vi "NavbalLabVIEW(15-5-28.vi"() -> ()   [LabVIEW 2012] (continued)
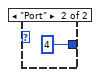
[diagram p2: hidden frame]
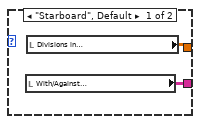
[diagram p4: hidden frame]
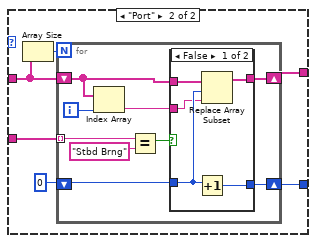
[diagram p6: hidden frame]
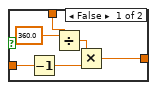
[diagram p10: hidden frame]
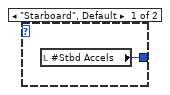
[diagram p11: hidden frame]
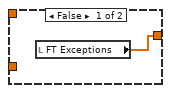
[diagram p12: hidden frame]
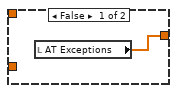
[diagram p13: hidden frame]
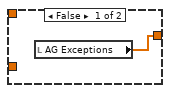
[diagram p14: hidden frame]
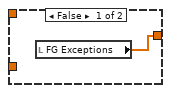
[diagram p15: hidden frame]
                  n2652 = Select(t=w3012, s=w3013, f="  ") -> (s? t:f=w3022:string)
                  n2653 = Number To Fractional String(number=w3057, precision (6)=i16 3) -> (F-format string=w3055:string[][])  [unwired: 2 in]
                  n2654 = Build Array(w3052, w3052, w3052, w3052) -> (w3054:string[])
                  n2655 = Select(t=w3044, s=w3036, f=w3020) -> (s? t:f=w3047:string)
                  n2656 = Select(t=w3044, s=w3037, f=w3022) -> (s? t:f=w3046:string)
                  n2657 = Select(t=w3044, s=w3038, f=w3024) -> (s? t:f=w3045:string)
                  n2658 = Insert Into Array(array=w3055, index (row)=1, new element=w3054) -> (w3051:string[][])  [unwired: 1 in]
                  n2659 = Replace Array Subset(array=w3051, new element=w3052, index (row)=3 ("disabled index (row)"), index (col)=0 ("disabled index (col)")) -> (w3042:string[][])
                  n2660 = Build Array(w3047, "  ", w3046, w3045) -> (w3043:string[])
                  n2661 = Insert Into Array(array=w3042, index (col)=4 ("disabled index (col)"), new element=w3043) -> (w3003:string[][])  [unwired: 1 in]
                  n2662 = property on="Aft Generator Balance Plane Split Options" class="MCListbox (strict)"("ItemNames"=w3003) -> ()  [unwired: 2 in, 2 out]
                  "AG Correction 1" <- w2995
                  "AG Correction 2B" <- w2994
                  "AG Correction 2A" <- w2993
                }
                frame 3 {
                  w3081 = 3 ("disabled index (col)")
                  w3091 = 3 ("disabled index (col)")
                  w3108 = 3 ("disabled index (col)")
                  w3121 = "Occupied!  "
                  w3129 = "  "
                  # "List box formatting"
                  n2663 = Build Array "Mass, angle, loc"(w3075, w3074, w3077) -> (w3139:T3)
                  n2664 = Build Array "Mass,angle, loc"(w3073, w3141, w3078) -> (w3140:T3)
                  n2665 = Build Array (concatenate)(w3140, w3139) -> (w3138:T3)
                  n2666 = Build Array "Percent,mass,angle,location"(w3142, w3070, w3143, w3079) -> (w3135:T3)
                  n2667 = Decrement(x=w3078) -> (x-1=w3116:dbl)
                  n2668 = Decrement(x=w3079) -> (x-1=w3115:dbl)
                  n2669 = Decrement(x=w3077) -> (x-1=w3117:dbl)
                  n2670 = Multiply(x=w3116, y=w3068) -> (x*y=w3090:dbl)
                  n2671 = Multiply(x=w3115, y=w3068) -> (x*y=w3080:dbl)
                  n2672 = Multiply(x=w3117, y=w3068) -> (x*y=w3109:dbl)
                  n2673 = Build Array (concatenate) "Percent"(w3137, w3138) -> (w3133:T3)
                  n2674 = Index Array(array=w3111, index (row)=w3080, index (col)=w3081) -> (element=w3112:bool)
                  n2675 = Index Array(array=w3111, index (row)=w3090, index (col)=w3091) -> (element=w3113:bool)
                  n2676 = Index Array(array=w3111, index (row)=w3109, index (col)=w3108) -> (element=w3114:bool)
                  n2677 = Index Array(array=w3076, index (row)=w3090, index (col)=w3091) -> (element=w3092:dbl)
                  n2678 = Index Array(array=w3076, index (row)=w3109, index (col)=w3108) -> (element=w3105:dbl)
                  n2679 = Index Array(array=w3076, index (row)=w3080, index (col)=w3081) -> (element=w3087:dbl)
                  n2680 = Greater Than 0?(x=w3092) -> (x > 0?=w3089:bool)
                  n2681 = Greater Than 0?(x=w3105) -> (x > 0?=w3106:bool)
                  n2682 = Greater Than 0?(x=w3087) -> (x > 0?=w3083:bool)
                  n2683 = Number To Fractional String(number=w3092, precision (6)=i16 1) -> (F-format string=w3093:string)  [unwired: 2 in]
                  n2684 = Number To Fractional String(number=w3105, precision (6)=i16 1) -> (F-format string=w3104:string)  [unwired: 2 in]
                  n2685 = Number To Fractional String(number=w3087, precision (6)=i16 1) -> (F-format string=w3086:string)  [unwired: 2 in]
                  n2686 = Concatenate Strings(w3093, " wt in hole") -> (w3088:string)
                  n2687 = Concatenate Strings(w3104, " wt in hole") -> (w3102:string)
                  n2688 = Concatenate Strings(w3086, " wt in hole") -> (w3082:string)
                  n2689 = Build Array (concatenate)(w3135, w3133) -> (w3134:T3)
                  n2690 = Select(t=w3082, s=w3083, f="  ") -> (s? t:f=w3096:string)
                  n2691 = Select(t=w3102, s=w3106, f="  ") -> (s? t:f=w3100:string)
                  n2692 = Select(t=w3088, s=w3089, f="  ") -> (s? t:f=w3098:string)
                  n2693 = Number To Fractional String(number=w3134, precision (6)=i16 3) -> (F-format string=w3132:string[][])  [unwired: 2 in]
                  n2694 = Build Array(w3129, w3129, w3129, w3129) -> (w3131:string[])
                  n2695 = Select(t=w3121, s=w3112, f=w3096) -> (s? t:f=w3124:string)
                  n2696 = Select(t=w3121, s=w3113, f=w3098) -> (s? t:f=w3123:string)
                  n2697 = Select(t=w3121, s=w3114, f=w3100) -> (s? t:f=w3122:string)
                  n2698 = Insert Into Array(array=w3132, index (row)=1, new element=w3131) -> (w3128:string[][])  [unwired: 1 in]
                  n2699 = Replace Array Subset(array=w3128, new element=w3129, index (row)=3 ("disabled index (row)"), index (col)=0 ("disabled index (col)")) -> (w3119:string[][])
                  n2700 = Build Array(w3124, "  ", w3123, w3122) -> (w3120:string[])
                  n2701 = Insert Into Array(array=w3119, index (col)=4 ("disabled index (col)"), new element=w3120) -> (w3118:string[][])  [unwired: 1 in]
                  n2702 = property on="Fwd Generator Balance Plane Split Options" class="MCListbox (strict)"("ItemNames"=w3118) -> ()  [unwired: 2 in, 2 out]
                  "FG Correction 1" <- w3069
                  "FG Correction 2A" <- w3072
                  "FG Correction 2B" <- w3071
                }
              }
            }
            "2wt-Exceptions" <- w2654
          }
        }
        n2703 = local read "AT Exceptions"() -> (w621:csg[])
        n2704 = local read "2wt-Exceptions"() -> (w620:csg[])
        n2705 = case shown="True" "Omit AT" {
          tunnel: w621 -> [_ w839]
          tunnel: w620 -> [_ w837]
          tunnel: [w833 w834] -> w619
          frame False {
            n2706 = local read "AT Exceptions"() -> (w833:csg[])
          }
          frame True {
            n2707 = Index Array(array=w837, index=0) -> (element=w835:csg)
            n2708 = Insert Into Array(array=w839, index=0, new element=w835) -> (w834:csg[])
          }
        }
        "AT Exceptions" <- w619
        n2709 = local read "FT Exceptions"() -> (w615:csg[])
        n2710 = local read "2wt-Exceptions"() -> (w616:csg[])
        n2711 = case shown="True" "Omit FT" {
          tunnel: w615 -> [_ w832]
          tunnel: w616 -> [_ w830]
          tunnel: [w826 w827] -> w617
          frame False {
            n2712 = local read "FT Exceptions"() -> (w826:csg[])
          }
          frame True {
            n2713 = Index Array(array=w830, index=1) -> (element=w828:csg)
            n2714 = Insert Into Array(array=w832, index=0, new element=w828) -> (w827:csg[])
          }
        }
        "FT Exceptions" <- w617
        n2715 = local read "AG Exceptions"() -> (w623:csg[])
        n2716 = local read "2wt-Exceptions"() -> (w624:csg[])
        n2717 = case shown="True" "Omit AG" {
          tunnel: w623 -> [_ w846]
          tunnel: w624 -> [_ w844]
          tunnel: [w840 w841] -> w625
          frame False {
            n2718 = local read "AG Exceptions"() -> (w840:csg[])
          }
          frame True {
            n2719 = Index Array(array=w844, index=2) -> (element=w842:csg)
            n2720 = Insert Into Array(array=w846, index=0, new element=w842) -> (w841:csg[])
          }
        }
        "AG Exceptions" <- w625
        n2721 = local read "FG Exceptions"() -> (w628:csg[])
        n2722 = local read "2wt-Exceptions"() -> (w627:csg[])
        n2723 = case shown="True" "Omit FG" {
          tunnel: w628 -> [_ w853]
          tunnel: w627 -> [_ w851]
          tunnel: [w847 w848] -> w626
          frame False {
            n2724 = local read "FG Exceptions"() -> (w847:csg[])
          }
          frame True {
            n2725 = Index Array(array=w851, index=3) -> (element=w849:csg)
            n2726 = Insert Into Array(array=w853, index=0, new element=w849) -> (w848:csg[])
          }
        }
        "FG Exceptions" <- w626
        n2727 = local read "Divisions in\nEach Plane"() -> (w636:T3)
        n2728 = local read "1st Available"() -> (w650:bool)
        n2729 = local read "2nd Available"() -> (w649:bool)
        n2730 = local read "3rd Available"() -> (w648:bool)
        n2731 = local read "4th Available"() -> (w647:bool)
        n2732 = case shown="True" w650 {
          tunnel: w636 -> [_ w1024]
          frame False {
          }
          frame True {
            n2733 = invoke on="Aft Turbine Balance Plane Split Options" class="MCListbox (strict)" method="Get DblClk Row"() -> ("Get Double-clicked Row"=w1025:i32)  [unwired: 3 in, 2 out]
            n2734 = Index Array(array=w1024, index (row)=0, index (col)=0 ("disabled index (col)")) -> (element=w1022:dbl)
            n2735 = case shown="2" w1025 {
              tunnel: w1022 -> [_ w1026 w1053]
              frame -2, Default {
                # "-2 is the variable value when no box is currently double clicked"
              }
              frame 0 {
                w1030 = 360.0 ("x")
                w1042 = 0 ("disabled index (col)")
                w1046 = 0 ("disabled index (col)")
                # "Update Pending weights Boolean Array\nwith selected split's locations"
                # "Update Inputs for Prediction tab\nto reflect selected weight split"
                # "Pull mass, Phase, and Location Data\nfrom listbox's array"
                # "Single Mass Option Selected"
                n2736 = local read "AT Correction 1"() -> (w1040:cdb)
                n2737 = Complex To Polar(r * e^(i*theta)=w1040) -> (r=w1039:dbl, theta=w1027:dbl)
                n2738 = Divide(x=w1027, y=3.141592653589793) -> (x/y=w1038:dbl)
                n2739 = local read "Correction Mag"() -> (w1047:T3)
                n2740 = Multiply ("Multiply.vi")(x=180.0, y=w1038) -> (x*y=w1033:dbl)
                n2741 = Add ("Add.vi")(x=w1033, y=w1030) -> (x+y=w1034:dbl)
                n2742 = Greater Than 0?(x=w1033) -> (x > 0?=w1035:bool)
                n2743 = Select(t=w1033, s=w1035, f=w1034) -> (s? t:f=w1032:dbl)
                n2744 = Divide(x=w1026, y=w1030) -> (x/y=w1031:dbl)
                n2745 = Replace Array Subset(array=w1047, new element=w1039, index (row)=w1046, index (col)=w1046) -> (w1045:T3)
                n2746 = Multiply ("Multiply.vi")(x=w1032, y=w1031) -> (x*y=w1029:dbl)
                n2747 = Increment(x=w1029) -> (x+1=w1028:dbl)
                n2748 = local read "Correction Loc"() -> (w1044:T3)
                n2749 = local write "Correction Mag"(w1045) -> ()
                n2750 = Replace Array Subset(array=w1044, new element=w1028, index (row)=w1042, index (col)=w1042) -> (w1043:T3)
                n2751 = local write "Correction Loc"(w1043) -> ()
                n2752 = property on="Aft Turbine Balance Plane Split Options" class="MCListbox (strict)"("SelColor"=u32 40727) -> ()  [unwired: 2 in, 2 out]
              }
              frame 2 {
                w1052 = 360.0 ("x")
                w1066 = 0 ("disabled index (col)")
                w1070 = 0 ("disabled index (col)")
                n2753 = local read "AT Correction 2A"() -> (w1048:cdb)
                n2754 = local read "AT Correction 2B"() -> (w1049:cdb)
                n2755 = local read "Correction Mag"() -> (w1071:T3)
                n2756 = Add ("Add.vi")(x=w1048, y=w1049) -> (x+y=w1065:cdb)
                n2757 = Complex To Polar ("Complex To Polar.vi")(r * e^(i*theta)=w1065) -> (r=w1064:dbl, theta=w1060:dbl)
                n2758 = Divide(x=w1060, y=3.141592653589793) -> (x/y=w1063:dbl)
                n2759 = Replace Array Subset(array=w1071, new element=w1064, index (row)=w1070, index (col)=w1070) -> (w1069:T3)
                n2760 = local write "Correction Mag"(w1069) -> ()
                n2761 = Multiply ("Multiply.vi")(x=180.0, y=w1063) -> (x*y=w1056:dbl)
                n2762 = local read "Correction Loc"() -> (w1068:T3)
                n2763 = Add ("Add.vi")(x=w1056, y=w1052) -> (x+y=w1057:dbl)
                n2764 = Greater Than 0?(x=w1056) -> (x > 0?=w1058:bool)
                n2765 = Select(t=w1056, s=w1058, f=w1057) -> (s? t:f=w1055:dbl)
                n2766 = Divide(x=w1053, y=w1052) -> (x/y=w1054:dbl)
                n2767 = Multiply ("Multiply.vi")(x=w1055, y=w1054) -> (x*y=w1051:dbl)
                n2768 = Increment(x=w1051) -> (x+1=w1050:dbl)
                n2769 = Replace Array Subset(array=w1068, new element=w1050, index (row)=w1066, index (col)=w1066) -> (w1067:T3)
                n2770 = local write "Correction Loc"(w1067) -> ()
                n2771 = property on="Aft Turbine Balance Plane Split Options" class="MCListbox (strict)"("SelColor"=u32 40727) -> ()  [unwired: 2 in, 2 out]
              }
            }
          }
        }
        n2772 = case shown="True" w649 {
          tunnel: w636 -> [_ w1073]
          frame False {
          }
          frame True {
            n2773 = invoke on="Fwd Turbine Balance Plane Split Options" class="MCListbox (strict)" method="Get DblClk Row"() -> ("Get Double-clicked Row"=w1076:i32)  [unwired: 3 in, 2 out]
            n2774 = Index Array(array=w1073, index (row)=1, index (col)=0 ("disabled index (col)")) -> (element=w1072:dbl)
            n2775 = case shown="0" w1076 {
              tunnel: w1072 -> [_ w1078 w1103]
              frame -2, Default {
              }
              frame 0 {
                w1084 = 360.0 ("x")
                n2776 = local read "FT Correction 1"() -> (w1082:cdb)
                n2777 = Complex To Polar(r * e^(i*theta)=w1082) -> (r=w1081:dbl, theta=w1077:dbl)
                n2778 = Divide(x=w1077, y=3.141592653589793) -> (x/y=w1092:dbl)
                n2779 = Multiply ("Multiply.vi")(x=180.0, y=w1092) -> (x*y=w1087:dbl)
                n2780 = Add ("Add.vi")(x=w1087, y=w1084) -> (x+y=w1088:dbl)
                n2781 = Divide(x=w1078, y=w1084) -> (x/y=w1085:dbl)
                n2782 = Greater Than 0?(x=w1087) -> (x > 0?=w1089:bool)
                n2783 = Select(t=w1087, s=w1089, f=w1088) -> (s? t:f=w1086:dbl)
                n2784 = local read "Correction Mag"() -> (w1100:T3)
                n2785 = local read "Correction Loc"() -> (w1097:T3)
                n2786 = Multiply ("Multiply.vi")(x=w1086, y=w1085) -> (x*y=w1083:dbl)
                n2787 = Increment(x=w1083) -> (x+1=w1079:dbl)
                n2788 = Replace Array Subset(array=w1097, new element=w1079, index (row)=1 ("disabled index (row)"), index (col)=0 ("disabled index (col)")) -> (w1096:T3)
                n2789 = Replace Array Subset(array=w1100, new element=w1081, index (row)=1 ("disabled index (row)"), index (col)=0 ("disabled index (col)")) -> (w1098:T3)
                n2790 = local write "Correction Loc"(w1096) -> ()
                n2791 = local write "Correction Mag"(w1098) -> ()
                n2792 = property on="Fwd Turbine Balance Plane Split Options" class="MCListbox (strict)"("SelColor"=u32 40727) -> ()  [unwired: 2 in, 2 out]
              }
              frame 2 {
                w1106 = 360.0 ("x")
                n2793 = local read "FT Correction 2A"() -> (w1102:cdb)
                n2794 = local read "FT Correction 2B"() -> (w1101:cdb)
                n2795 = Add(x=w1102, y=w1101) -> (x+y=w1120:cdb)
                n2796 = Complex To Polar(r * e^(i*theta)=w1120) -> (r=w1119:dbl, theta=w1115:dbl)
                n2797 = local read "Correction Mag"() -> (w1126:T3)
                n2798 = Divide(x=w1115, y=3.141592653589793) -> (x/y=w1118:dbl)
                n2799 = Multiply ("Multiply.vi")(x=180.0, y=w1118) -> (x*y=w1109:dbl)
                n2800 = local read "Correction Loc"() -> (w1123:T3)
                n2801 = Add(x=w1109, y=w1106) -> (x+y=w1110:dbl)
                n2802 = Replace Array Subset(array=w1126, new element=w1119, index (row)=1 ("disabled index (row)"), index (col)=0 ("disabled index (col)")) -> (w1124:T3)
                n2803 = Greater Than 0?(x=w1109) -> (x > 0?=w1111:bool)
                n2804 = local write "Correction Mag"(w1124) -> ()
                n2805 = Select(t=w1109, s=w1111, f=w1110) -> (s? t:f=w1105:dbl)
                n2806 = Divide(x=w1103, y=w1106) -> (x/y=w1107:dbl)
                n2807 = Multiply ("Multiply.vi")(x=w1105, y=w1107) -> (x*y=w1108:dbl)
                n2808 = Increment(x=w1108) -> (x+1=w1104:dbl)
                n2809 = Replace Array Subset(array=w1123, new element=w1104, index (row)=1 ("disabled index (row)"), index (col)=0 ("disabled index (col)")) -> (w1122:T3)
                n2810 = local write "Correction Loc"(w1122) -> ()
                n2811 = property on="Fwd Turbine Balance Plane Split Options" class="MCListbox (strict)"("SelColor"=u32 40727) -> ()  [unwired: 2 in, 2 out]
              }
            }
          }
        }
        n2812 = case shown="True" w648 {
          tunnel: w636 -> [_ w1128]
          frame False {
          }
          frame True {
            n2813 = invoke on="Aft Generator Balance Plane Split Options" class="MCListbox (strict)" method="Get DblClk Row"() -> ("Get Double-clicked Row"=w1131:i32)  [unwired: 3 in, 2 out]
            n2814 = Index Array(array=w1128, index (row)=2, index (col)=0 ("disabled index (col)")) -> (element=w1127:dbl)
            n2815 = case shown="2" w1131 {
              tunnel: w1127 -> [_ w1133 w1157]
              frame -2, Default {
              }
              frame 0 {
                w1143 = 360.0 ("x")
                n2816 = local read "AG Correction 1"() -> (w1146:cdb)
                n2817 = Complex To Polar(r * e^(i*theta)=w1146) -> (r=w1145:dbl, theta=w1134:dbl)
                n2818 = Divide(x=w1134, y=3.141592653589793) -> (x/y=w1135:dbl)
                n2819 = Multiply ("Multiply.vi")(x=180.0, y=w1135) -> (x*y=w1140:dbl)
                n2820 = Greater Than 0?(x=w1140) -> (x > 0?=w1138:bool)
                n2821 = local read "Correction Mag"() -> (w1155:T3)
                n2822 = Add ("Add.vi")(x=w1140, y=w1143) -> (x+y=w1139:dbl)
                n2823 = Select(t=w1140, s=w1138, f=w1139) -> (s? t:f=w1141:dbl)
                n2824 = Divide(x=w1133, y=w1143) -> (x/y=w1142:dbl)
                n2825 = Multiply ("Multiply.vi")(x=w1141, y=w1142) -> (x*y=w1144:dbl)
                n2826 = Increment(x=w1144) -> (x+1=w1132:dbl)
                n2827 = Replace Array Subset(array=w1155, new element=w1145, index (row)=2 ("disabled index (row)"), index (col)=0 ("disabled index (col)")) -> (w1153:T3)
                n2828 = local read "Correction Loc"() -> (w1152:T3)
                n2829 = local write "Correction Mag"(w1153) -> ()
                n2830 = Replace Array Subset(array=w1152, new element=w1132, index (row)=2 ("disabled index (row)"), index (col)=0 ("disabled index (col)")) -> (w1151:T3)
                n2831 = local write "Correction Loc"(w1151) -> ()
                n2832 = property on="Aft Generator Balance Plane Split Options" class="MCListbox (strict)"("SelColor"=u32 40727) -> ()  [unwired: 2 in, 2 out]
              }
              frame 2 {
                w1156 = 360.0 ("x")
                n2833 = local read "AG Correction 2A"() -> (w1159:cdb)
                n2834 = local read "AG Correction 2B"() -> (w1158:cdb)
                n2835 = Add(x=w1159, y=w1158) -> (x+y=w1175:cdb)
                n2836 = Complex To Polar(r * e^(i*theta)=w1175) -> (r=w1174:dbl, theta=w1170:dbl)
                n2837 = local read "Correction Mag"() -> (w1181:T3)
                n2838 = Divide(x=w1170, y=3.141592653589793) -> (x/y=w1173:dbl)
                n2839 = Multiply ("Multiply.vi")(x=180.0, y=w1173) -> (x*y=w1164:dbl)
                n2840 = Add(x=w1164, y=w1156) -> (x+y=w1165:dbl)
                n2841 = Greater Than 0?(x=w1164) -> (x > 0?=w1166:bool)
                n2842 = local read "Correction Loc"() -> (w1178:T3)
                n2843 = Select(t=w1164, s=w1166, f=w1165) -> (s? t:f=w1161:dbl)
                n2844 = Replace Array Subset(array=w1181, new element=w1174, index (row)=2 ("disabled index (row)"), index (col)=0 ("disabled index (col)")) -> (w1179:T3)
                n2845 = Divide(x=w1157, y=w1156) -> (x/y=w1163:dbl)
                n2846 = local write "Correction Mag"(w1179) -> ()
                n2847 = Multiply ("Multiply.vi")(x=w1161, y=w1163) -> (x*y=w1162:dbl)
                n2848 = Increment(x=w1162) -> (x+1=w1160:dbl)
                n2849 = Replace Array Subset(array=w1178, new element=w1160, index (row)=2 ("disabled index (row)"), index (col)=0 ("disabled index (col)")) -> (w1177:T3)
                n2850 = local write "Correction Loc"(w1177) -> ()
                n2851 = property on="Aft Generator Balance Plane Split Options" class="MCListbox (strict)"("SelColor"=u32 40727) -> ()  [unwired: 2 in, 2 out]
              }
            }
          }
        }
        n2852 = case shown="True" w647 {
          tunnel: w636 -> [_ w1183]
          frame False {
          }
          frame True {
            n2853 = invoke on="Fwd Generator Balance Plane Split Options" class="MCListbox (strict)" method="Get DblClk Row"() -> ("Get Double-clicked Row"=w1186:i32)  [unwired: 3 in, 2 out]
            n2854 = Index Array(array=w1183, index (row)=2, index (col)=0 ("disabled index (col)")) -> (element=w1182:dbl)
            n2855 = case shown="2" w1186 {
              tunnel: w1182 -> [_ w1191 w1212]
              frame -2, Default {
              }
              frame 0 {
                w1193 = 360.0 ("x")
                n2856 = local read "FG Correction 1"() -> (w1190:cdb)
                n2857 = Complex To Polar(r * e^(i*theta)=w1190) -> (r=w1189:dbl, theta=w1188:dbl)
                n2858 = Divide(x=w1188, y=3.141592653589793) -> (x/y=w1201:dbl)
                n2859 = Multiply ("Multiply.vi")(x=180.0, y=w1201) -> (x*y=w1196:dbl)
                n2860 = local read "Correction Mag"() -> (w1210:T3)
                n2861 = Add ("Add.vi")(x=w1196, y=w1193) -> (x+y=w1197:dbl)
                n2862 = Greater Than 0?(x=w1196) -> (x > 0?=w1198:bool)
                n2863 = Select(t=w1196, s=w1198, f=w1197) -> (s? t:f=w1195:dbl)
                n2864 = Divide(x=w1191, y=w1193) -> (x/y=w1194:dbl)
                n2865 = Multiply ("Multiply.vi")(x=w1195, y=w1194) -> (x*y=w1192:dbl)
                n2866 = Increment(x=w1192) -> (x+1=w1187:dbl)
                n2867 = Replace Array Subset(array=w1210, new element=w1189, index (row)=3 ("disabled index (row)"), index (col)=0 ("disabled index (col)")) -> (w1208:T3)
                n2868 = local read "Correction Loc"() -> (w1207:T3)
                n2869 = local write "Correction Mag"(w1208) -> ()
                n2870 = Replace Array Subset(array=w1207, new element=w1187, index (row)=3 ("disabled index (row)"), index (col)=0 ("disabled index (col)")) -> (w1206:T3)
                n2871 = local write "Correction Loc"(w1206) -> ()
                n2872 = property on="Fwd Generator Balance Plane Split Options" class="MCListbox (strict)"("SelColor"=u32 40727) -> ()  [unwired: 2 in, 2 out]
              }
              frame 2 {
                w1215 = 360.0 ("x")
                n2873 = local read "FG Correction 2A"() -> (w1225:cdb)
                n2874 = local read "FG Correction 2B"() -> (w1224:cdb)
                n2875 = Add(x=w1225, y=w1224) -> (x+y=w1230:cdb)
                n2876 = Complex To Polar(r * e^(i*theta)=w1230) -> (r=w1229:dbl, theta=w1213:dbl)
                n2877 = local read "Correction Mag"() -> (w1236:T3)
                n2878 = Divide(x=w1213, y=3.141592653589793) -> (x/y=w1223:dbl)
                n2879 = Multiply ("Multiply.vi")(x=180.0, y=w1223) -> (x*y=w1218:dbl)
                n2880 = Greater Than 0?(x=w1218) -> (x > 0?=w1220:bool)
                n2881 = Add ("Add.vi")(x=w1218, y=w1215) -> (x+y=w1219:dbl)
                n2882 = Divide(x=w1212, y=w1215) -> (x/y=w1216:dbl)
                n2883 = Select(t=w1218, s=w1220, f=w1219) -> (s? t:f=w1217:dbl)
                n2884 = Replace Array Subset(array=w1236, new element=w1229, index (row)=3 ("disabled index (row)"), index (col)=0 ("disabled index (col)")) -> (w1234:T3)
                n2885 = local read "Correction Loc"() -> (w1233:T3)
                n2886 = Multiply ("Multiply.vi")(x=w1217, y=w1216) -> (x*y=w1214:dbl)
                n2887 = local write "Correction Mag"(w1234) -> ()
                n2888 = Increment(x=w1214) -> (x+1=w1211:dbl)
                n2889 = Replace Array Subset(array=w1233, new element=w1211, index (row)=3 ("disabled index (row)"), index (col)=0 ("disabled index (col)")) -> (w1232:T3)
                n2890 = property on="Fwd Generator Balance Plane Split Options" class="MCListbox (strict)"("SelColor"=u32 40727) -> ()  [unwired: 2 in, 2 out]
                n2891 = local write "Correction Loc"(w1232) -> ()
              }
            }
          }
        }
      }
    }
    n2892 = case "Refresh Run Name Listbox on Import Mag-Phase Tab" shown="True" w348 {
      tunnel: w363 -> [_ w461]
      tunnel: w359 -> [_ w460]
      tunnel: "Select Side to Analyze" -> [_ w379]
      frame False {
      }
      frame True {
        w404 = sgl[] []  # Empty Array
        w409 = sgl[] []  # Empty Array
        w414 = sgl[] []  # Empty Array
        w421 = sgl[] []  # Empty Array
        w458 = sgl[] []  # Empty Array
        # "2. Use every other\ncolumn"
        # "1. Choose first\nthree rows"
        n2893 = call <vilib>:"New Report.vi"("report type"=T11."Excel", "template (empty)"=w461) -> ("report out"=w434:refnum<class "NI_report.lvclass">, "error out"=w433:errorcluster)  [unwired: 12 in]
        n2894 = call <vilib>:"Excel Get Worksheet.vi"("report in"=w434, "worksheet index (0)"=w460, "error in (no error)"=w433) -> ("report out"=w536:refnum<class "NI_report.lvclass">, "error out"=w535:errorcluster)  [unwired: 11 out]
        n2895 = call <vilib>:"Excel Get Worksheet.vi"("report in"=w434, "worksheet index (0)"=1, "error in (no error)"=w433) -> ("report out"=w512:refnum<class "NI_report.lvclass">, "error out"=w511:errorcluster)  [unwired: 11 out]
        n2896 = local read "Weight Category FT"() -> (w495:u16)
        n2897 = call <vilib>:"Excel Get Worksheet.vi"("report in"=w434, "worksheet index (0)"=1, "error in (no error)"=w433) -> ("report out"=w456:refnum<class "NI_report.lvclass">, "error out"=w457:errorcluster)  [unwired: 11 out]
        n2898 = call-poly <vilib>:"Excel Get Data.vi"("report in"=w512, "data type"=string[][] [], "start (-1, -1)"=cluster{"row":i32, "column":i32} {"row"=0, "column"=0}, "end (-1, -1)"=cluster{"row":i32, "column":i32} {"row"=0, "column"=15} ("start (-1, -1)"), "error in (no error)"=w511) -> ("data"=w507:string[][])  [unwired: 10 out]
        n2899 = call <vilib>:"Excel Get Last Row.vi"("report in"=w456, "error in (no error)"=w457) -> ("report out"=w454:refnum<class "NI_report.lvclass">, "MS Office parameters out"=w455:T14, "error out"=w453:errorcluster)  [unwired: 11 in]
        n2900 = Increment(x="No. Runs") -> (x+1=w500:i32)
        n2901 = Multiply(x=w500, y=2) -> (x*y=w502:i32)
        n2902 = Index Array(array=w507, index (row)=0) -> (element=w505:string[])  [unwired: 1 in]
        n2903 = Unbundle(w455) -> ("position (Excel)"=w493:cluster{"row":i32, "column":i32})  [unwired: 2 out]
        n2904 = Bundle("row"=2, w502) -> (w501:cluster{"row":i32, i32})  [unwired: 1 in]
        n2905 = call-poly <vilib>:"Excel Get Data.vi"("report in"=w536, "data type"=string[][] [], "start (-1, -1)"=cluster{"row":i32, "column":i32} {"row"=0, "column"=1}, "end (-1, -1)"=w501, "error in (no error)"=w535) -> ("data"=w514:string[][])  [unwired: 10 out]
        n2906 = Transpose 2D Array(2D array=w514) -> (transposed array=w531:string[][])
        n2907 = Unbundle(w493) -> ("row"=w494:i32)  [unwired: 1 out]
        n2908 = Bundle(1, "Weight Category FT"=w495) -> (w492:cluster{i32, "Weight Category FT":u16})  [unwired: 1 in]
        n2909 = property on="Weight Category AT" class="Ring (strict)"("Strings []"=w505) -> ()  [unwired: 2 in, 2 out]
        n2910 = Bundle("row"=w494, "Weight Category FT"=w495) -> (w496:cluster{"row":i32, "Weight Category FT":u16})  [unwired: 1 in]
        n2911 = call-poly <vilib>:"Excel Get Data.vi"("report in"=w454, "data type"=sgl[][] [], "start (-1, -1)"=w492, "end (-1, -1)"=w496, "error in (no error)"=w453) -> ("data"=w498:dbl[][])  [unwired: 10 out]
        n2912 = Index Array(array=w498, index (col)=0 ("disabled index (col)")) -> (element=w416:dbl[])  [unwired: 1 in]
        n2913 = for {
          shift-right: [w554] -> w420
          shift-left: w421 -> [w555]
          tunnel: w416 -> [w553] mode=indexing
          n2914 = Build Array (concatenate)(w555, w553) -> (w554:dbl[])
        }
        n2915 = Insert Into Array(array=w420, index=0, new element=0 ("new element/subarray")) -> (w417:dbl[])
        n2916 = Index Array(array=w531, index (col)=1 ("disabled index (col)")) -> (element=w530:string[])  [unwired: 1 in]
        n2917 = Index Array(array=w531, index (col)=2 ("disabled index (col)")) -> (element=w529:string[])  [unwired: 1 in]
        n2918 = Index Array(array=w531, index (col)=0 ("disabled index (col)")) -> (element=w516:string[])  [unwired: 1 in]
        n2919 = Sort 1D Array(array=w417) -> (sorted array=→"FT Weights":dbl[])
        n2920 = Decimate 1D Array(w516) -> (w513:string[])  [unwired: 1 out]
        n2921 = Decimate 1D Array(w529) -> (w524:string[])  [unwired: 1 out]
        n2922 = Decimate 1D Array(w530) -> (w526:string[])  [unwired: 1 out]
        n2923 = Array Size(array=w513) -> (size(s)=w515:i32)
        n2924 = property on="Weight Category FT" class="Ring (strict)"("Strings []"=w505) -> ()  [unwired: 2 in, 2 out]
        n2925 = Reshape Array(w524, w515, 1 ("dimension size")) -> (w518:string[][])
        n2926 = Reshape Array(w513, w515, 1 ("dimension size")) -> (w523:string[][])
        n2927 = Reshape Array(w526, w515, 1 ("dimension size")) -> (w521:string[][])
        n2928 = property on="Start Point:" class="Ring (strict)"("Strings []"=w513) -> ()  [unwired: 2 in, 2 out]
        n2929 = Insert Into Array(array=w523, index (col)=1 ("disabled index (col)"), new element=w521) -> (w519:string[][])  [unwired: 1 in]
        n2930 = local read "Weight Category AG"() -> (w485:u16)
        n2931 = property on="Weight Category AG" class="Ring (strict)"("Strings []"=w505) -> ()  [unwired: 2 in, 2 out]
        n2932 = Insert Into Array(array=w519, index (col)=2 ("disabled index (col)"), new element=w518) -> (w517:string[][])  [unwired: 1 in]
        n2933 = property on="Multicolumn Listbox" class="MCListbox (strict)"("ItemNames"=w517) -> ()  [unwired: 2 in, 2 out]
        n2934 = Unbundle(w455) -> ("position (Excel)"=w483:cluster{"row":i32, "column":i32})  [unwired: 2 out]
        n2935 = property on="Weight Category FG" class="Ring (strict)"("Strings []"=w505) -> ()  [unwired: 2 in, 2 out]
        n2936 = Unbundle(w483) -> ("row"=w484:i32)  [unwired: 1 out]
        n2937 = Bundle(1, "Weight Category AG"=w485) -> (w482:cluster{i32, "Weight Category AG":u16})  [unwired: 1 in]
        n2938 = Bundle("row"=w484, "Weight Category AG"=w485) -> (w486:cluster{"row":i32, "Weight Category AG":u16})  [unwired: 1 in]
        n2939 = call-poly <vilib>:"Excel Get Data.vi"("report in"=w454, "data type"=sgl[][] [], "start (-1, -1)"=w482, "end (-1, -1)"=w486, "error in (no error)"=w453) -> ("data"=w488:dbl[][])  [unwired: 10 out]
        n2940 = Index Array(array=w488, index (col)=0 ("disabled index (col)")) -> (element=w396:dbl[])  [unwired: 1 in]
        n2941 = for {
          shift-right: [w551] -> w411
          shift-left: w414 -> [w552]
          tunnel: w396 -> [w550] mode=indexing
          n2942 = Build Array (concatenate)(w552, w550) -> (w551:dbl[])
        }
        n2943 = Insert Into Array(array=w411, index=0, new element=0 ("new element/subarray")) -> (w410:dbl[])
        n2944 = Sort 1D Array(array=w410) -> (sorted array=→"AG Weights":dbl[])
        n2945 = local write "AT Exceptions"(w458) -> ()
        n2946 = local write "FT Exceptions"(w458) -> ()
        n2947 = local write "AG Exceptions"(w458) -> ()
        n2948 = local write "FG Exceptions"(w458) -> ()
        n2949 = local read "Weight Category FG"() -> (w476:u16)
        n2950 = case shown="\"Port\"" w379 {
          tunnel: [w541 w543] -> w378
          tunnel: [w540 w542] -> w377
          frame "Starboard", Default {
            n2951 = local read "With/Against\nRotation S"() -> (w540:string[][])
            n2952 = local read "Divisions in\nEach Plane S"() -> (w541:T3)
          }
          frame "Port" {
            n2953 = local read "Divisions in\nEach Plane P"() -> (w543:T3)
            n2954 = local read "With/Against\nRotation P"() -> (w542:string[][])
          }
        }
        n2955 = Unbundle(w455) -> ("position (Excel)"=w474:cluster{"row":i32, "column":i32})  [unwired: 2 out]
        n2956 = local write "Divisions in\nEach Plane"(w378) -> ()
        n2957 = local write "With/Against\nRotation"(w377) -> ()
        n2958 = Unbundle(w474) -> ("row"=w475:i32)  [unwired: 1 out]
        n2959 = Bundle(1, "Weight Category FG"=w476) -> (w473:cluster{i32, "Weight Category FG":u16})  [unwired: 1 in]
        n2960 = Bundle("row"=w475, "Weight Category FG"=w476) -> (w477:cluster{"row":i32, "Weight Category FG":u16})  [unwired: 1 in]
        n2961 = call-poly <vilib>:"Excel Get Data.vi"("report in"=w454, "data type"=sgl[][] [], "start (-1, -1)"=w473, "end (-1, -1)"=w477, "error in (no error)"=w453) -> ("data"=w478:dbl[][])  [unwired: 10 out]
        n2962 = Index Array(array=w478, index (col)=0 ("disabled index (col)")) -> (element=w398:dbl[])  [unwired: 1 in]
        n2963 = for {
          shift-right: [w548] -> w406
          shift-left: w409 -> [w549]
          tunnel: w398 -> [w547] mode=indexing
          n2964 = Build Array (concatenate)(w549, w547) -> (w548:dbl[])
        }
        n2965 = Insert Into Array(array=w406, index=0, new element=0 ("new element/subarray")) -> (w405:dbl[])
        n2966 = Sort 1D Array(array=w405) -> (sorted array=→"FG Weights":dbl[])
        n2967 = local read "Sensor Info"() -> (w426:string[][])
        n2968 = local read "Weight Category AT"() -> (w467:u16)
        n2969 = Index Array(array=w426, index (col)=0 ("disabled index (col)")) -> (element=w429:string[])  [unwired: 1 in]
        n2970 = Index Array(array=w426, index (col)=2 ("disabled index (col)")) -> (element=w425:string[])  [unwired: 1 in]
        n2971 = case shown="\"Starboard\", Default" w379 {
          tunnel: w429 -> [w560 w582]
          tunnel: [w558 w580] -> w424
          tunnel: w425 -> [w559 w581]
          tunnel: [w556 w578] -> w423
          frame "Starboard", Default {
            n2972 = Array Size(array=w560) -> (size(s)=w561:i32)
            n2973 = for {
              N: w561 -> [_]
              tunnel: w559 -> [w570] mode=indexing
              shift-right: [w567] -> w558
              shift-left: w560 -> [w564]
              shift-right: [w565] -> w556
              shift-left: 0 -> [w566]
              i -> [w563]
              n2974 = Index Array(array=w564, index=w563) -> (element=w562:string)
              n2975 = Equal?(x=w570, y="Port Brng") -> (x = y?=w568:bool)
              n2976 = case shown="False" w568 {
                tunnel: [w574 w577] -> w567
                tunnel: w564 -> [w575 w577]
                tunnel: w566 -> [w572 w576]
                tunnel: [w573 w576] -> w565
                tunnel: w562 -> [w571 _]
                frame False {
                  n2977 = Increment(x=w572) -> (x+1=w573:i32)
                  n2978 = Replace Array Subset(array=w575, new element=w571, index=w572) -> (w574:string[])
                }
                frame True {
                }
              }
            }
          }
          frame "Port" {
            n2979 = Array Size(array=w582) -> (size(s)=w583:i32)
            n2980 = for {
              N: w583 -> [_]
              tunnel: w581 -> [w592] mode=indexing
              shift-right: [w589] -> w580
              shift-left: w582 -> [w586]
              shift-right: [w587] -> w578
              shift-left: 0 -> [w588]
              i -> [w585]
              n2981 = Index Array(array=w586, index=w585) -> (element=w584:string)
              n2982 = Equal?(x=w592, y="Stbd Brng") -> (x = y?=w590:bool)
              n2983 = case shown="False" w590 {
                tunnel: [w596 w599] -> w589
                tunnel: w586 -> [w597 w599]
                tunnel: w588 -> [w594 w598]
                tunnel: [w595 w598] -> w587
                tunnel: w584 -> [w593 _]
                frame False {
                  n2984 = Increment(x=w594) -> (x+1=w595:i32)
                  n2985 = Replace Array Subset(array=w597, new element=w593, index=w594) -> (w596:string[])
                }
                frame True {
                }
              }
            }
          }
        }
        n2986 = Unbundle(w455) -> ("position (Excel)"=w465:cluster{"row":i32, "column":i32})  [unwired: 2 out]
        n2987 = Unbundle(w465) -> ("row"=w466:i32)  [unwired: 1 out]
        n2988 = Bundle(1, "Weight Category AT"=w467) -> (w464:cluster{i32, "Weight Category AT":u16})  [unwired: 1 in]
        n2989 = Bundle("row"=w466, "Weight Category AT"=w467) -> (w468:cluster{"row":i32, "Weight Category AT":u16})  [unwired: 1 in]
        n2990 = call-poly <vilib>:"Excel Get Data.vi"("report in"=w454, "data type"=sgl[][] [], "start (-1, -1)"=w464, "end (-1, -1)"=w468, "error in (no error)"=w453) -> ("data"=w470:dbl[][])  [unwired: 10 out]
        n2991 = Index Array(array=w470, index (col)=0 ("disabled index (col)")) -> (element=w395:dbl[])  [unwired: 1 in]
        n2992 = for {
          shift-right: [w545] -> w401
          shift-left: w404 -> [w546]
          tunnel: w395 -> [w544] mode=indexing
          n2993 = Build Array (concatenate)(w546, w544) -> (w545:dbl[])
        }
        n2994 = Insert Into Array(array=w401, index=0, new element=0 ("new element/subarray")) -> (w400:dbl[])
        n2995 = Sort 1D Array(array=w400) -> (sorted array=→"AT Weights":dbl[])
        n2996 = Reshape Array(w424, w423) -> (→"Sensor Column":string[])
        n2997 = call <vilib>:"Excel Get Worksheet.vi"("report in"=w434, "worksheet index (0)"=2, "error in (no error)"=w433) -> ("report out"=w382:refnum<class "NI_report.lvclass">, "error out"=w381:errorcluster)  [unwired: 11 out]
        n2998 = call <vilib>:"Excel Get Last Row.vi"("report in"=w382, "error in (no error)"=w381) -> ("report out"=w451:refnum<class "NI_report.lvclass">, "MS Office parameters out"=w448:T14, "error out"=w450:errorcluster)  [unwired: 11 in]
        n2999 = Unbundle(w448) -> ("position (Excel)"=w449:cluster{"row":i32, "column":i32})  [unwired: 2 out]
        n3000 = call-poly <vilib>:"Excel Get Data.vi"("report in"=w382, "data type"=sgl[][] [], "start (-1, -1)"=cluster{"start row":i32, "start column":i32} {"start row"=3, "start column"=0} ("start (0, 0)"), "end (-1, -1)"=cluster{"start row":i32, "start column":i32} {"start row"=4, "start column"=0} ("start (0, 0)"), "error in (no error)"=w381) -> ("data"=w386:dbl[][])  [unwired: 10 out]
        n3001 = Unbundle(w449) -> ("row"=w439:i32)  [unwired: 1 out]
        n3002 = Index Array(array=w386, index (row)=1, index (col)=0) -> (element=w385:dbl)
        n3003 = Index Array(array=w386, index (row)=0, index (col)=0) -> (element=w384:dbl)
        n3004 = Subtract(x=w439, y=2.0) -> (x-y=w431:dbl)
        n3005 = Bundle("row"=w439, "start column"=8) -> (w444:cluster{"row":i32, "start column":i32})  [unwired: 1 in]
        n3006 = call-poly <vilib>:"Excel Get Data.vi"("report in"=w451, "data type"=sgl[][] [], "start (-1, -1)"=cluster{"start row":i32, "start column":i32} {"start row"=3, "start column"=1} ("start (0, 0)"), "end (-1, -1)"=w444, "error in (no error)"=w450) -> ("data"=w435:dbl[][])  [unwired: 10 out]
        n3007 = Subtract(x=w385, y=w384) -> (x-y=w383:dbl)
        n3008 = Reciprocal(x=w383) -> (1/x=w380:dbl)
        n3009 = Array Subset(array=w435, index (row)=0 ("index"), length (row)=w431, index (col)=0 ("index"), length (col)=4 ("length")) -> (w442:dbl[][])
        n3010 = Array Subset(array=w435, index (row)=0 ("index"), length (row)=w431, index (col)=4 ("index"), length (col)=4 ("length")) -> (w436:dbl[][])
        n3011 = property on="Holes/Division" class="DigNum (strict)"("Value"=w380) -> ()  [unwired: 2 in, 2 out]
        n3012 = local write "Existing Plane Wts Port"(w442) -> ()
        n3013 = local write "Existing Plane Wts Stbd"(w436) -> ()
        "DataTab" <- w460
      }
    }
  }
